vi "ORM Full Example.vi"() -> ()   [LabVIEW 2020, in "ORM_Examples.lvlib"]
uses:
  ORM_Examples.lvlib
  syslogs/syslogcluster.ctl
  syslogs/type.ctl
  <vilib>/Viviota/shared/ORM.lvlibp/ORM/SqlMapper/SqlMapper.lvclass
  <vilib>/Viviota/shared/ORM.lvlibp/ORM/TypeMap/TypeMap.lvclass
  syslogs/syslogs.lvclass
  syslogs/syslogs.lvclass/syslogs.ctl
  05764d67-500d-4b48-8229-7f30afda64a9.vi
  <vilib>/numeric/Random Number (Range) DBL.vi
  6377c067-cfd4-4b32-8915-bdbb0adddf30.vi
  0386ddb9-f275-45d1-b7b4-687382315ca8.vi
  9e31a9a6-021b-445f-b77c-036ae0c99ecd.vi
  80d51cb0-5371-4b91-9bea-091f0997292c.vi
  4f43362e-f8cc-419c-9351-c2ae03d92930.vi
  4ebe4bd5-e54f-48a5-86b4-46e7f1bb6f5a.vi
  0437fd30-8bf0-43ae-9868-d75e91ee3b4b.vi
  c0336298-bb8b-4fb9-a827-d7aab42547a5.vi
  syslogs/Write id.vi
  syslogs/Write type.vi
  b6464032-c044-4b29-b6c1-8ea3cc686848.vi
  98a8b6ed-17aa-439b-9f56-f47df0604604.vi
  05764d67-500d-4b48-8229-7f30afda64a9.vi/bd23ee19-7bd1-410a-a455-250ae7eff562.vi
  6377c067-cfd4-4b32-8915-bdbb0adddf30.vi/35b31214-e0d6-4ae0-b34c-13eba9df70db.vi
  6377c067-cfd4-4b32-8915-bdbb0adddf30.vi/2e8f1eab-5a58-47e6-9224-d0a2895e31fd.vi
  0386ddb9-f275-45d1-b7b4-687382315ca8.vi/35b31214-e0d6-4ae0-b34c-13eba9df70db.vi
  0386ddb9-f275-45d1-b7b4-687382315ca8.vi/2e8f1eab-5a58-47e6-9224-d0a2895e31fd.vi
  9e31a9a6-021b-445f-b77c-036ae0c99ecd.vi/a9ccc3c9-891a-4d80-8d4f-837bdef88ccd.vi
  9e31a9a6-021b-445f-b77c-036ae0c99ecd.vi/8216614f-f413-45b3-8111-14f8d0271ea5.vi
  9e31a9a6-021b-445f-b77c-036ae0c99ecd.vi/fc6a5c23-d21f-4d2c-895e-66da96fa9491.vi
  80d51cb0-5371-4b91-9bea-091f0997292c.vi/a9ccc3c9-891a-4d80-8d4f-837bdef88ccd.vi
  80d51cb0-5371-4b91-9bea-091f0997292c.vi/8216614f-f413-45b3-8111-14f8d0271ea5.vi
  80d51cb0-5371-4b91-9bea-091f0997292c.vi/fc6a5c23-d21f-4d2c-895e-66da96fa9491.vi
  4f43362e-f8cc-419c-9351-c2ae03d92930.vi/a9ccc3c9-891a-4d80-8d4f-837bdef88ccd.vi
  4f43362e-f8cc-419c-9351-c2ae03d92930.vi/8216614f-f413-45b3-8111-14f8d0271ea5.vi
  4f43362e-f8cc-419c-9351-c2ae03d92930.vi/fc6a5c23-d21f-4d2c-895e-66da96fa9491.vi
  4ebe4bd5-e54f-48a5-86b4-46e7f1bb6f5a.vi/ce8babb2-619c-4b95-b634-e027cd54a13e.vi
  4ebe4bd5-e54f-48a5-86b4-46e7f1bb6f5a.vi/383c36e0-7191-4c70-923d-4cc1411f3794.vi
  4ebe4bd5-e54f-48a5-86b4-46e7f1bb6f5a.vi/dcffdf9a-60b2-440f-af14-9d618c05381d.vi
  0437fd30-8bf0-43ae-9868-d75e91ee3b4b.vi/ce8babb2-619c-4b95-b634-e027cd54a13e.vi
  0437fd30-8bf0-43ae-9868-d75e91ee3b4b.vi/383c36e0-7191-4c70-923d-4cc1411f3794.vi
  0437fd30-8bf0-43ae-9868-d75e91ee3b4b.vi/dcffdf9a-60b2-440f-af14-9d618c05381d.vi
  c0336298-bb8b-4fb9-a827-d7aab42547a5.vi/ce8babb2-619c-4b95-b634-e027cd54a13e.vi
  c0336298-bb8b-4fb9-a827-d7aab42547a5.vi/383c36e0-7191-4c70-923d-4cc1411f3794.vi
  c0336298-bb8b-4fb9-a827-d7aab42547a5.vi/dcffdf9a-60b2-440f-af14-9d618c05381d.vi
  b6464032-c044-4b29-b6c1-8ea3cc686848.vi/93c2cd5d-a53a-4cc2-b8c3-9c3eef6598b6.vi
  98a8b6ed-17aa-439b-9f56-f47df0604604.vi/bd23ee19-7bd1-410a-a455-250ae7eff562.vi
  9e31a9a6-021b-445f-b77c-036ae0c99ecd.vi/fc6a5c23-d21f-4d2c-895e-66da96fa9491.vi/9d007ba8-e96f-4737-8d8a-6b46cf7f5c4a.vi
  9e31a9a6-021b-445f-b77c-036ae0c99ecd.vi/fc6a5c23-d21f-4d2c-895e-66da96fa9491.vi/050765a8-e5d4-4415-b637-62775228e838.vi
  80d51cb0-5371-4b91-9bea-091f0997292c.vi/fc6a5c23-d21f-4d2c-895e-66da96fa9491.vi/9d007ba8-e96f-4737-8d8a-6b46cf7f5c4a.vi
  80d51cb0-5371-4b91-9bea-091f0997292c.vi/fc6a5c23-d21f-4d2c-895e-66da96fa9491.vi/050765a8-e5d4-4415-b637-62775228e838.vi
  4f43362e-f8cc-419c-9351-c2ae03d92930.vi/fc6a5c23-d21f-4d2c-895e-66da96fa9491.vi/9d007ba8-e96f-4737-8d8a-6b46cf7f5c4a.vi
  4f43362e-f8cc-419c-9351-c2ae03d92930.vi/fc6a5c23-d21f-4d2c-895e-66da96fa9491.vi/050765a8-e5d4-4415-b637-62775228e838.vi
  <vilib>/Viviota/shared/ORM_ADONet.lvlibp/ADOMapper/ADOMapper.lvclass
  C:/Program Files/National Instruments/LabVIEW 2024/vi.lib/Viviota/shared/ORM.lvlibp/ORM/SqlMapper/SqlMapper.lvclass
  <vilib>/Viviota/shared/ORM.lvlibp/ORM/TypeMap/Write Autokey.vi
  <vilib>/Viviota/shared/ORM.lvlibp/ORM/TypeMap/Write Table Name.vi
  <vilib>/Viviota/shared/ORM_DBC_Sqlite.lvlibp/Sqlite Connect.vi
  <vilib>/Viviota/shared/ORM_DBC_Npgsql.lvlibp/Postgresql Connect.vi
  <vilib>/Viviota/shared/ORM_DBC_Mssql.lvlibp/SQL Connect.vi
  <vilib>/Utility/error.llb/Error Cluster From Error Code.vi
  <vilib>/Viviota/shared/ORM.lvlibp/ORM/TypeMap/Read TypeMap.vi
  <vilib>/Viviota/shared/ORM.lvlibp/ORM/SqlMapper/End Transaction.vi
  <vilib>/Viviota/shared/ORM.lvlibp/ORM/TypeMap/Where.vi
  <vilib>/Viviota/shared/ORM.lvlibp/ORM/Query Result/Next.vi
  <vilib>/Viviota/shared/ORM.lvlibp/ORM/TypeMap/ToLabVIEW_Wrap.vi
  <vilib>/Viviota/shared/ORM.lvlibp/ORM/DynamicParameters/DynamicParameters.lvclass
  <vilib>/Viviota/shared/ORM.lvlibp/ORM/Query Result/Query Result.lvclass
  ORM_API/ORM_API.lvlib
  <vilib>/Viviota/shared/ORM_ADONet.lvlibp
  <vilib>/Viviota/shared/ORM_DBC_Sqlite.lvlibp/DBC.lvclass
  <vilib>/Viviota/shared/ORM_DBC_Mssql.lvlibp/DBC.lvclass
  <vilib>/Viviota/shared/ORM_DBC_Npgsql.lvlibp/DBC.lvclass
  <vilib>/Viviota/shared/ORM.lvlibp/Transaction Logger/Log Map/LogMap.lvclass
  baf2aaaf-5c25-4d5a-81b7-a781a1585a2d.vi
  84ec28b1-c7a7-454f-ae3a-af914e71003c.vi
  50dc8464-3f00-4ac1-a87d-782bf5ccae4b.vi
  C:/Program Files/National Instruments/LabVIEW 2024/vi.lib/Viviota/shared/ORM_ADONet.lvlibp/ADOMapper/ADOMapper.lvclass
panel:
  out "DeleteTime":dbl
  in  "DeleteId":i32
  in  "DeleteEntry":bool
  out "QueryTime":dbl
  out "Count":i32
  out "ResultsTable":string
  out "Results":T1[](array[typedef]) {"Time Stamp" format="%<%x %.3X>T"}
  in  "limit":i32=10
  in  "ReturnAll":bool=TRUE
  in  "WHERE mode":enum32{"id", "type", "where"}(radio)=enum."type"
  in  "ExecuteQuery":bool
  in  "Explicit WHERE clause":string="executiontime < 4 AND executiontime > 2"
  in  "SyslogId":i32
  in  "SyslogType":string="warning"
  out "lastId":i32
  out "CreateTime":dbl
  in  "Use Bulk Create":bool=TRUE
  in  "Records":i32=100
  in  "PopulateTable":bool
  out "Error Out":errorcluster
  in  "Close":bool
  in  "DeleteTable":bool
  in  "CreateTable":bool
  in  "ConnectionString":string
  in  "SQLite Path":path
  in  "Connect":bool
  in  "DbType":string(combo)="Sqlite"
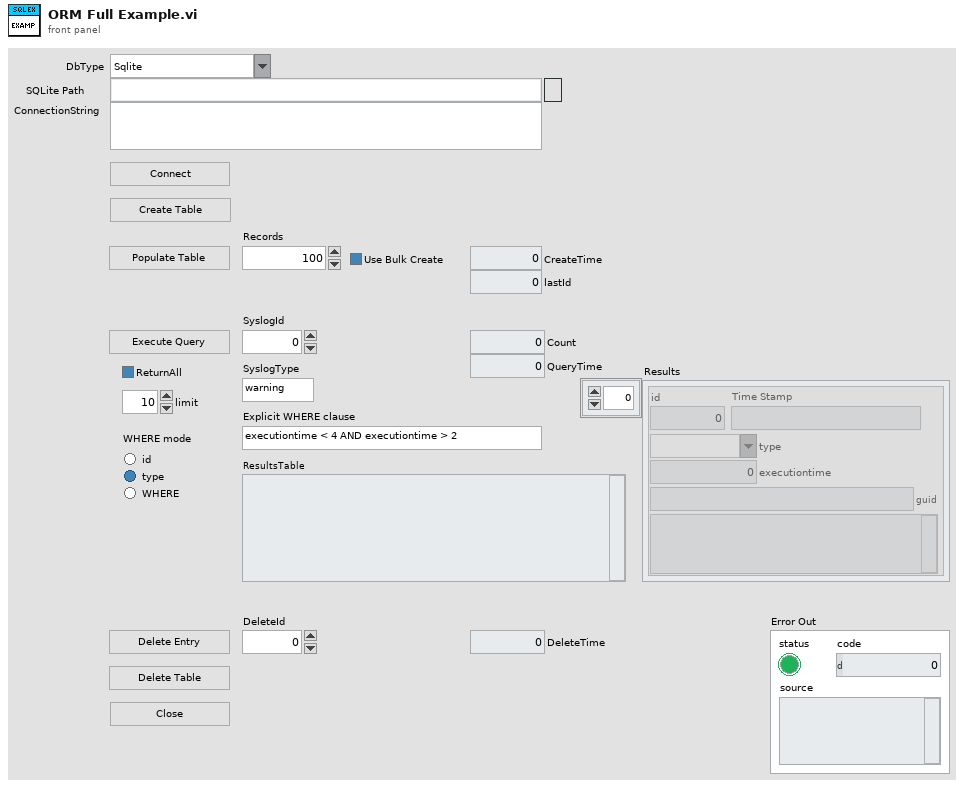
[diagram p1: front panel]
types:
  T1 = typedef "ORM_Examples.lvlib/syslogs.lvclass/syslogcluster.ctl" = cluster{"id":i32, "type":T2, "executiontime":dbl, "log":string, "guid":string, "Time Stamp":timestamp}
  T2 = typedef "ORM_Examples.lvlib/syslogs.lvclass/type.ctl" = string
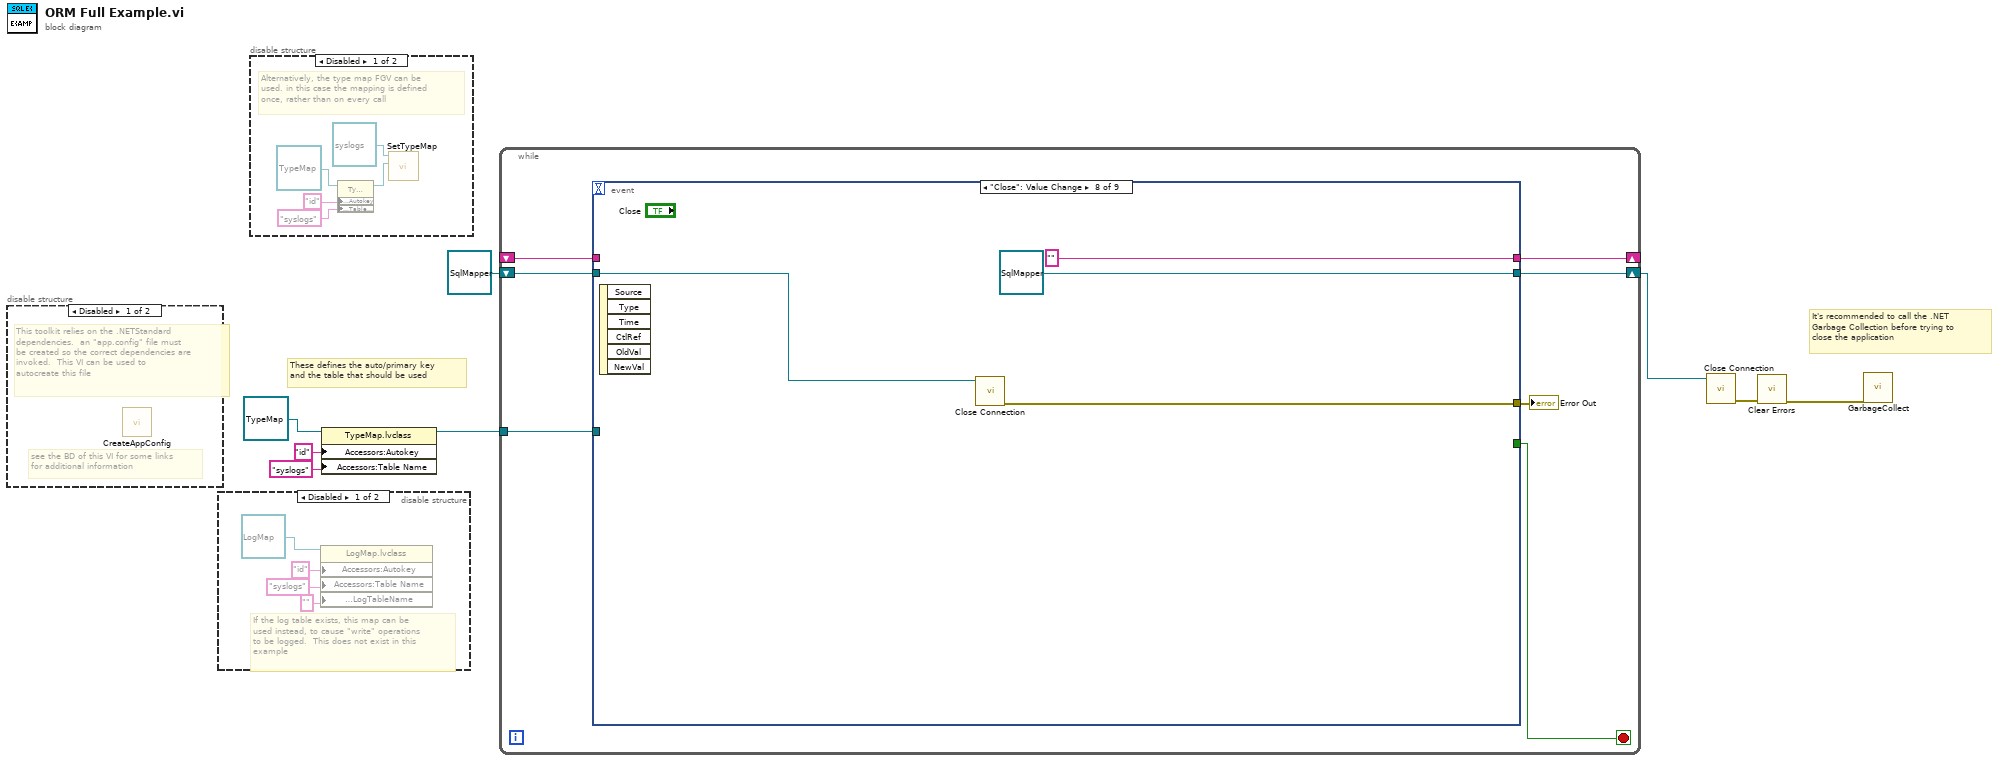
[diagram p0: block diagram]
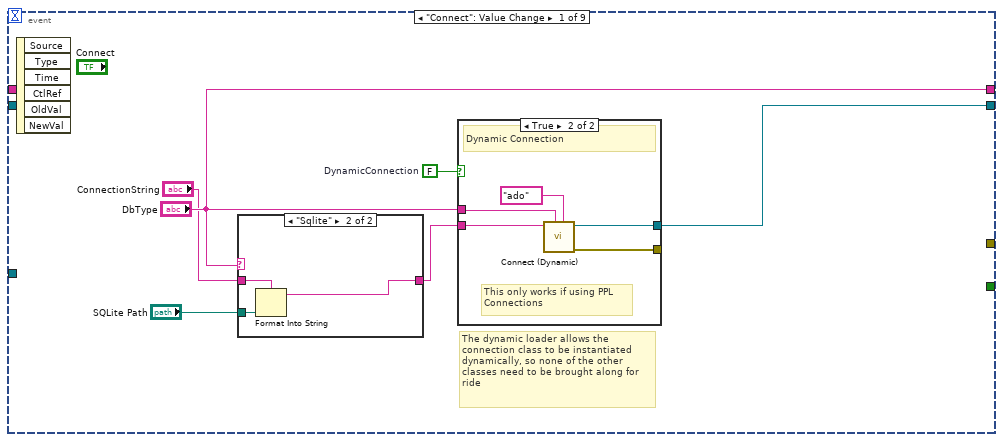
[diagram p5: hidden frame]
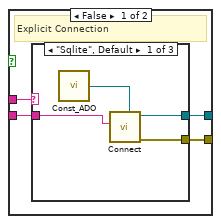
[diagram p7: hidden frame]
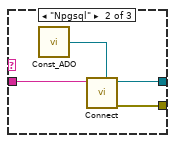
[diagram p8: hidden frame]
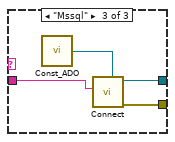
[diagram p9: hidden frame]
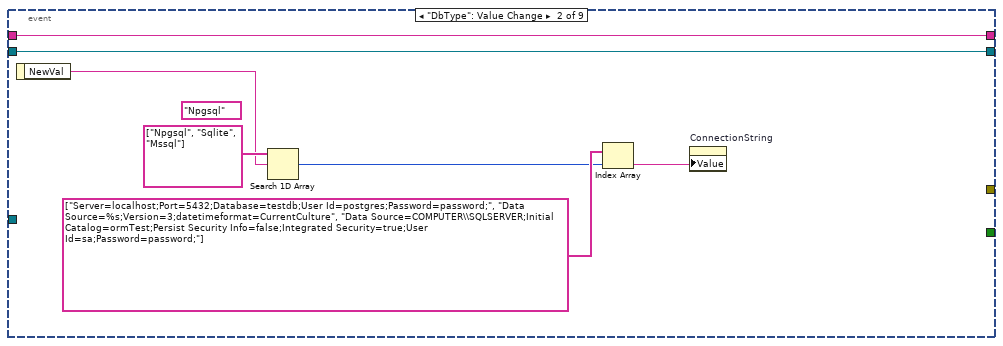
[diagram p10: hidden frame]
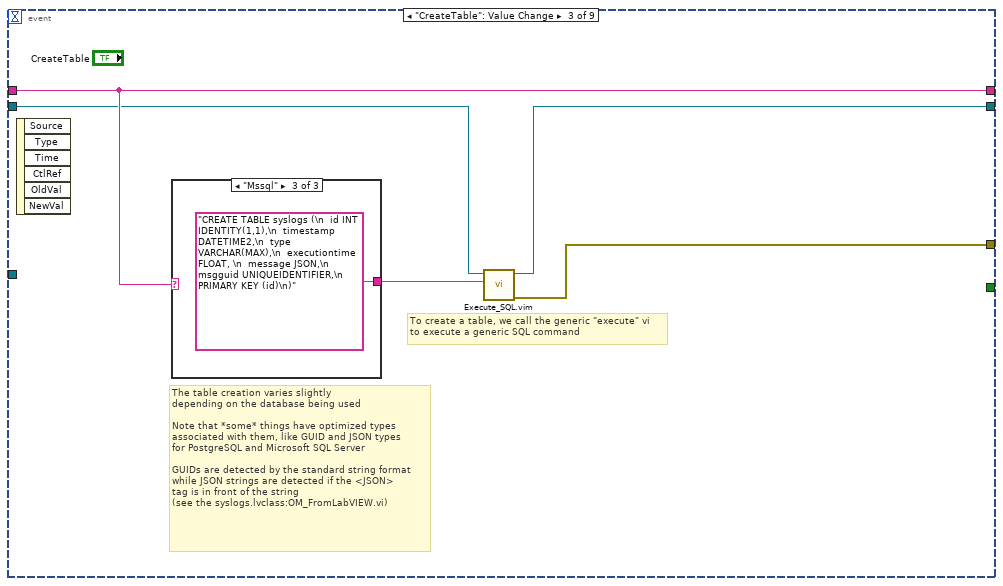
[diagram p11: hidden frame]
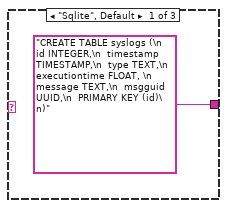
[diagram p12: hidden frame]
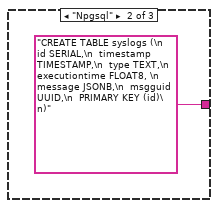
[diagram p13: hidden frame]
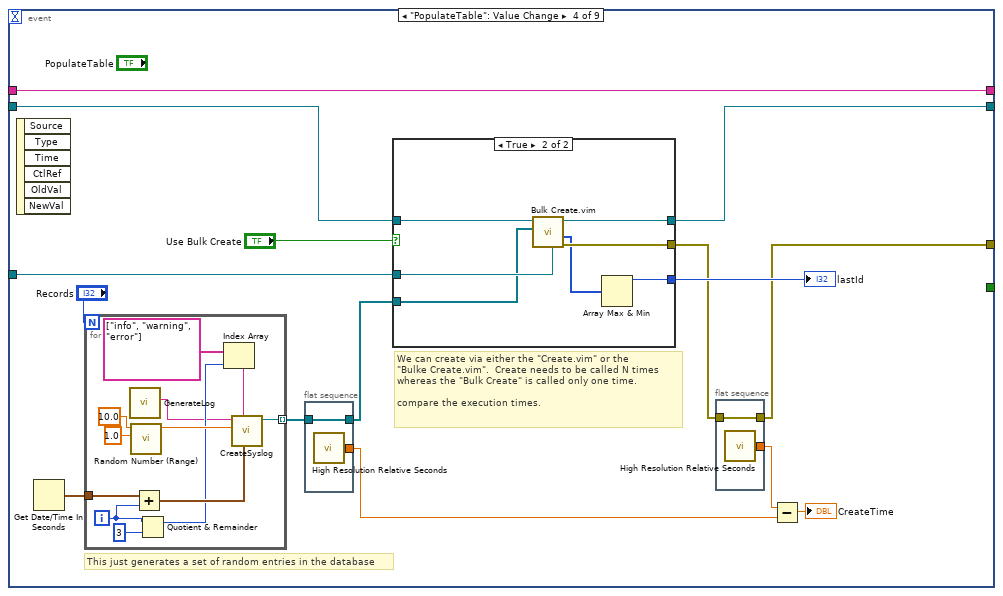
[diagram p14: hidden frame]
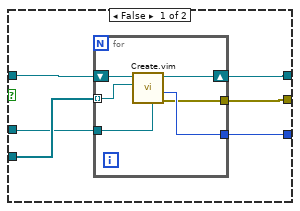
[diagram p15: hidden frame]
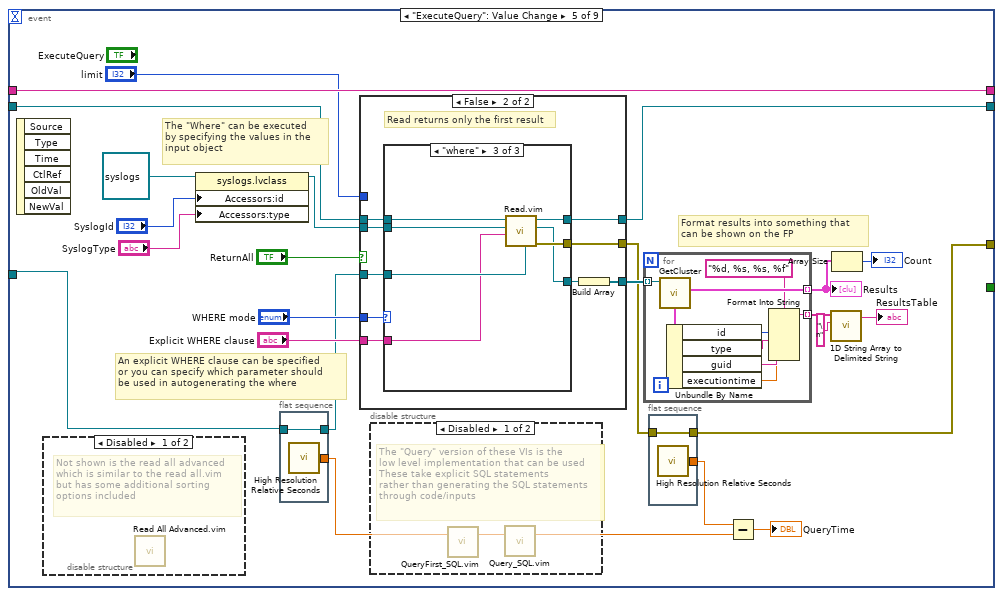
[diagram p16: hidden frame]
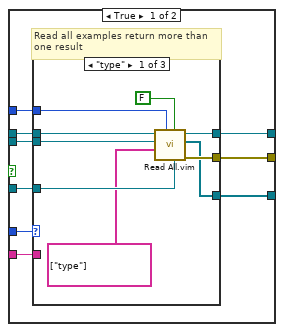
[diagram p19: hidden frame]
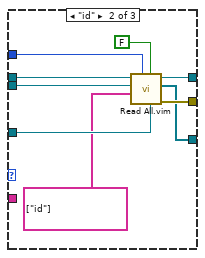
[diagram p20: hidden frame]
diagram:
  # "It's recommended to call the .NET \nGarbage Collection before trying to \nclose the application"
  # "These defines the auto/primary key\nand the table that should be used"
  n1 = disable-structure shown="Disabled" {
    frame Disabled {
      # "see the BD of this VI for some links\nfor additional information"
      # "This toolkit relies on the .NETStandard\ndependencies.  an \"app.config\" file must\nbe created so the correct dependencies are\ninvoked.  This VI can be used to \nautocreate this file"
      n2 = call "CreateAppConfig.vi"() -> ()  [unwired: 11 in, 1 out]
    }
    frame Enabled {
    }
  }
  n3 = disable-structure shown="Disabled" {
    frame Disabled {
      # "If the log table exists, this map can be\nused instead, to cause \"write\" operations\nto be logged.  This does not exist in this\nexample"
      n4 = property class="LogMap.lvclass"(reference=refnum<class "LogMap.lvclass"> refnum ("TypeMap in"), "Accessors:Autokey"="id" ("Autokey"), "Accessors:Table Name"="syslogs" ("Table Name"), "Data Member Access:LogTableName"="" ("LogTableName")) -> ()  [unwired: 1 in, 2 out]
    }
    frame Enabled {
    }
  }
  n5 = disable-structure shown="Disabled" {
    frame Disabled {
      # "Alternatively, the type map FGV can be\nused. in this case the mapping is defined\nonce, rather than on every call"
      n6 = property class="TypeMap.lvclass"(reference=refnum<class "TypeMap.lvclass"> refnum ("TypeMap in"), "Accessors:Autokey"="id" ("Autokey"), "Accessors:Table Name"="syslogs" ("Table Name")) -> (reference out=w14:refnum<class "TypeMap.lvclass">)  [unwired: 1 in, 1 out]
      n7 = call "SetTypeMap.vi"("TypeMap in"=w14, "object in"=refnum<class "syslogs.lvclass"> refnum ("ORM_Examples.lvlib:syslogs.lvclass")) -> ()  [unwired: 7 in, 3 out]
    }
    frame Enabled {
    }
  }
  n8 = property class="TypeMap.lvclass"(reference=refnum<class "TypeMap.lvclass"> refnum ("TypeMap in"), "Accessors:Autokey"="id" ("Autokey"), "Accessors:Table Name"="syslogs" ("Table Name")) -> (reference out=w4:refnum<class "TypeMap.lvclass">)  [unwired: 1 in, 1 out]
  n9 = while {
    shift-right: [w23] -> w3
    shift-left: refnum<class "SqlMapper.lvclass"> refnum ("SqlMapper out") -> [w22]
    shift-right: [w21] -> _
    shift-left: _ -> [w20]
    tunnel: w4 -> [w18]
    stop <- w24 stop-if-true
    n10 = event shown="[7] \"Close\": Value Change" {
      selector: _ -> [_ _ _ _ _ _ _ _ _]
      dyn-events: _ -> [_ _ _ _ _ _ _ _ _]
      timeout: _ -> [_ _ _ _ _ _ _ _ _]
      tunnel: [_ _ _ _ _ _ _ _ w251] -> w24
      tunnel: [w29 w56 w64 w82 w142 w233 w242 refnum<class "SqlMapper.lvclass"> refnum ("SqlMapper out") w249] -> w23
      tunnel: w22 -> [_ w56 w66 w83 w143 w234 w243 w246 w249]
      tunnel: ["DbType" w61 w67 w85 w144 w235 w244 "" ("DbType") w250] -> w21
      tunnel: w20 -> [_ w61 w67 w85 w144 w235 w244 _ w250]
      tunnel: [_ _ w63 w75 w126 w226 w241 w245 _] -> w19
      tunnel: w18 -> [_ _ _ w84 w125 w229 _ _ _]
      event "Connect": Value Change {
        w30 = FALSE  # DynamicConnection
        # "The dynamic loader allows the \nconnection class to be instantiated\ndynamically, so none of the other\nclasses need to be brought along for\nride"
        n11 = event-data() -> ()  [unwired: 1 in, 6 out]
        n12 = case shown="\"Sqlite\"" "DbType" {
          tunnel: "ConnectionString" -> [w31 w34]
          tunnel: "SQLite Path" -> [_ w33]
          tunnel: [w31 w32] -> w25
          frame "False", Default {
          }
          frame "Sqlite" {
            n13 = Format Into String(format string=w34, w33) -> (resulting string=w32:string)  [unwired: 2 in, 1 out]
          }
        }
        n14 = case shown="True" w30 {
          tunnel: "DbType" -> [w38 w53]
          tunnel: [w37 w55] -> w29
          tunnel: [w36 w54] -> _
          tunnel: w25 -> [w35 w51]
          frame False {
            # "Explicit Connection"
            n15 = case shown="\"Sqlite\", Default" w38 {
              tunnel: [w40 w44 w49] -> w37
              tunnel: [w41 w45 w48] -> w36
              tunnel: w35 -> [w39 w43 w47]
              frame "Sqlite", Default {
                n16 = call <vilib>:"Const_ADO.vi"() -> ("ADOMapper"=w42:refnum<class "ADOMapper.lvclass">)
                n17 = call-poly "Connect.vi"("SqlMapper Type"=w42, "Connection String"=w39) -> ("error out"=w41:errorcluster, "SqlMapper out"=w40:refnum<class "ADOMapper.lvclass">)  [unwired: 8 in]
              }
              frame "Npgsql" {
                n18 = call <vilib>:"Const_ADO.vi"() -> ("ADOMapper"=w46:refnum<class "ADOMapper.lvclass">)
                n19 = call-poly "Connect.vi"("SqlMapper Type"=w46, "Connection String"=w43) -> ("error out"=w45:errorcluster, "SqlMapper out"=w44:refnum<class "ADOMapper.lvclass">)  [unwired: 8 in]
              }
              frame "Mssql" {
                n20 = call <vilib>:"Const_ADO.vi"() -> ("ADOMapper"=w50:refnum<class "ADOMapper.lvclass">)
                n21 = call-poly "Connect.vi"("SqlMapper Type"=w50, "Connection String"=w47) -> ("error out"=w48:errorcluster, "SQL Mapper"=w49:refnum<class "ADOMapper.lvclass">)  [unwired: 8 in]
              }
            }
          }
          frame True {
            # "This only works if using PPL\nConnections"
            # "Dynamic Connection"
            n22 = call "Connect (Dynamic).vi"("SqlMapper"="ado", "DbType"=w53, "Connection String"=w51) -> ("error out"=w54:errorcluster, "SqlMapper out"=w55:refnum<class "SqlMapper.lvclass">)  [unwired: 7 in]
          }
        }
      }
      event "DbType": Value Change {
        (unwired) "Npgsql" ("DbType")
        n23 = event-data() -> ("NewVal"=w57:string)  [unwired: 1 in]
        n24 = Search 1D Array(1D array=string[] ["Npgsql", "Sqlite", "Mssql"], element=w57) -> (index of element=w59:i32)  [unwired: 1 in]
        n25 = Index Array(array=string[] ["Server=localhost;Port=5432;Database=testdb;User Id=postgres;Password=password;", "Data Source=%s;Version=3;datetimeformat=CurrentCulture", "Data Source=COMPUTER\\SQLSERVER;Initial Catalog=ormTest;Persist Security Info=false;Integrated Security=true;User Id=sa;Password=password;"], index=w59) -> (element=w58:string)
        n26 = property on="ConnectionString" class="Str"("Value"=w58) -> ()  [unwired: 2 in, 2 out]
      }
      event "CreateTable": Value Change {
        # "The table creation varies slightly\ndepending on the database being used\n\nNote that *some* things have optimized types\nassociated with them, like GUID and JSON types\nfor PostgreSQL and Microsoft SQL Server\n\nGUIDs are detected by the standard string format\nwhile JSON strings are detected if the <JSON>\ntag is in front of the string \n(see the syslogs.lvclass:OM_FromLabVIEW.vi)"
        # "To create a table, we call the generic \"execute\" vi\nto execute a generic SQL command"
        n27 = event-data() -> ()  [unwired: 1 in, 6 out]
        n28 = case shown="\"Mssql\"" w67 {
          tunnel: ["CREATE TABLE syslogs (\n  id INTEGER,\n  timestamp TIMESTAMP,\n  type TEXT,\n  executiontime FLOAT, \n  message TEXT,\n  msgguid UUID,\n  PRIMARY KEY (id)\n)" "CREATE TABLE syslogs (\n  id SERIAL,\n  timestamp TIMESTAMP,\n  type TEXT,\n  executiontime FLOAT8, \n  message JSONB,\n  msgguid UUID,\n  PRIMARY KEY (id)\n)" "CREATE TABLE syslogs (\n  id INT IDENTITY(1,1),\n  timestamp DATETIME2,\n  type VARCHAR(MAX),\n  executiontime FLOAT, \n  message JSON,\n  msgguid UNIQUEIDENTIFIER,\n  PRIMARY KEY (id)\n)"] -> w65
          frame "Sqlite", Default {
          }
          frame "Npgsql" {
          }
          frame "Mssql" {
          }
        }
        n29 = call "Execute_SQL.vim"("sql"=w65, "SqlMapper in"=w66) -> ("error out"=w63:errorcluster, "SqlMapper out"=w64:refnum<class "SqlMapper.lvclass">)  [unwired: 7 in, 1 out]
      }
      event "PopulateTable": Value Change {
        # "We can create via either the \"Create.vim\" or the \n\"Bulke Create.vim\".  Create needs to be called N times\nwhereas the \"Bulk Create\" is called only one time.\n\ncompare the execution times."
        # "This just generates a set of random entries in the database"
        n30 = event-data() -> ()  [unwired: 1 in, 6 out]
        n31 = Get Date/Time In Seconds() -> (seconds since 1Jan1904=w81:timestamp)
        n32 = for {
          N: "Records" -> [_]
          tunnel: [w101] -> w78 mode=indexing
          tunnel: w81 -> [w97]
          i -> [w95]
          n33 = call "GenerateLog.vi"() -> ("JSON"=w90:string)  [unwired: 10 in, 1 out]
          n34 = call-poly <vilib>:"Random Number (Range).vi"("lower bound (0)"=1.0, "upper bound (100)"=10.0) -> ("number"=w98:dbl)  [unwired: 9 in]
          n35 = Add(x=w97, y=w95) -> (x+y=w96:timestamp)
          n36 = Quotient & Remainder(x=w95, y=3) -> (x-y*floor(x/y)=w92:i32)  [unwired: 1 out]
          n37 = Index Array(array=T2[] ["info", "warning", "error"] ("Array"), index=w92) -> (element=w91:T2)
          n38 = call "CreateSyslog.vi"("timestamp"=w96, "type"=w91, "executiontime"=w98, "log"=w90) -> ("syslog out"=w101:refnum<class "syslogs.lvclass">)  [unwired: 6 in, 1 out]
        }
        n39 = flat-sequence {
          tunnel: [w89] -> w73
          tunnel: w78 -> [w88]
          tunnel: [w88] -> w77
          frame #0 {
            n40 = call <vilib>:"High Resolution Relative Seconds.vi"() -> ("relative seconds"=w89:dbl)
          }
        }
        n41 = case shown="True" "Use Bulk Create" {
          tunnel: w84 -> [w102 w120]
          tunnel: [w104 w119] -> w76
          tunnel: w83 -> [w107 w118]
          tunnel: [w106 w117] -> w82
          tunnel: w77 -> [w103 w116]
          tunnel: [w105 w114] -> w80
          frame False {
            n42 = for {
              tunnel: [w111] -> w105
              tunnel: [w110] -> w104
              shift-right: [w112] -> w106
              shift-left: w107 -> [w113]
              tunnel: w103 -> [w109] mode=indexing
              tunnel: w102 -> [w108]
              n43 = call "Create.vim"("TypeMap in"=w108, "object in"=w109, "SqlMapper in"=w113) -> ("error out"=w110:errorcluster, "id"=w111:i32, "SqlMapper out"=w112:refnum<class "SqlMapper.lvclass">)  [unwired: 5 in, 1 out]
            }
          }
          frame True {
            n44 = call "Bulk Create.vim"("TypeMap in"=w120, "object in"=w116, "SqlMapper in"=w118) -> ("error out"=w119:errorcluster, "id"=w115:i32[], "SqlMapper out"=w117:refnum<class "SqlMapper.lvclass">)  [unwired: 5 in, 1 out]
            n45 = Array Max & Min(array=w115) -> (max value=w114:i32)  [unwired: 3 out]
          }
        }
        "lastId" <- w80
        n46 = flat-sequence {
          tunnel: [w87] -> w74
          tunnel: w76 -> [w86]
          tunnel: [w86] -> w75
          frame #0 {
            n47 = call <vilib>:"High Resolution Relative Seconds.vi"() -> ("relative seconds"=w87:dbl)
          }
        }
        n48 = Subtract(x=w74, y=w73) -> (x-y=→"CreateTime":dbl)
      }
      event "ExecuteQuery": Value Change {
        # "An explicit WHERE clause can be specified\nor you can specify which parameter should\nbe used in autogenerating the where"
        # "The \"Where\" can be executed\nby specifying the values in the \ninput object"
        # "Format results into something that \ncan be shown on the FP"
        n49 = event-data() -> ()  [unwired: 1 in, 6 out]
        n50 = disable-structure shown="Disabled" {
          frame Disabled {
            # "Not shown is the read all advanced\nwhich is similar to the read all.vim\nbut has some additional sorting\noptions included"
            n51 = call "Read All Advanced.vim"() -> ()  [unwired: 9 in, 3 out]
          }
          frame Enabled {
          }
        }
        n52 = property class="syslogs.lvclass"(reference=refnum<class "syslogs.lvclass"> refnum ("ORM_Examples.lvlib:syslogs.lvclass"), "Accessors:id"="SyslogId", "Accessors:type"="SyslogType") -> (reference out=w139:refnum<class "syslogs.lvclass">)  [unwired: 1 in, 1 out]
        n53 = flat-sequence {
          tunnel: [w148] -> w123
          tunnel: w125 -> [w147]
          tunnel: [w147] -> w124
          frame #0 {
            n54 = call <vilib>:"High Resolution Relative Seconds.vi"() -> ("relative seconds"=w148:dbl)
          }
        }
        n55 = case shown="False" "ReturnAll" {
          tunnel: w143 -> [w165 w201]
          tunnel: [w164 w200] -> w142
          tunnel: w124 -> [w163 w199]
          tunnel: [w162 w198] -> w127
          tunnel: "WHERE mode" -> [w161 w197]
          tunnel: w139 -> [w160 w196]
          tunnel: "Explicit WHERE clause" -> [w159 w195]
          tunnel: "limit" -> [w158 _]
          tunnel: [w157 w193] -> w134
          frame True {
            # "Read all examples return more than\none result"
            n56 = case shown="\"type\"" w161 {
              tunnel: w165 -> [w174 w183 w192]
              tunnel: [w173 w182 w191] -> w164
              tunnel: w163 -> [w172 w181 w190]
              tunnel: [w171 w180 w189] -> w162
              tunnel: w160 -> [w170 w179 w188]
              tunnel: w159 -> [_ _ w187]
              tunnel: [w168 w177 w186] -> w157
              tunnel: w158 -> [w167 w176 w185]
              frame "type" {
                n57 = call "Read All.vim"("TypeMap in"=w172, "Select All"=FALSE, "Limit"=w167, "WHERE"=string[] ["type"], "Object"=w170, "SqlMapper in"=w174) -> ("error out"=w171:errorcluster, "Query Results"=w168:refnum<class "syslogs.lvclass">[], "SqlMapper out"=w173:refnum<class "SqlMapper.lvclass">)  [unwired: 3 in]
              }
              frame "id" {
                n58 = call "Read All.vim"("TypeMap in"=w181, "Select All"=FALSE, "Limit"=w176, "WHERE"=string[] ["id"], "Object"=w179, "SqlMapper in"=w183) -> ("error out"=w180:errorcluster, "Query Results"=w177:refnum<class "syslogs.lvclass">[], "SqlMapper out"=w182:refnum<class "SqlMapper.lvclass">)  [unwired: 3 in]
              }
              frame "where" {
                n59 = call "Read All.vim"("TypeMap in"=w190, "Select All"=FALSE, "Limit"=w185, "WHERE"=w187, "Object"=w188, "SqlMapper in"=w192) -> ("error out"=w189:errorcluster, "Query Results"=w186:refnum<class "syslogs.lvclass">[], "SqlMapper out"=w191:refnum<class "SqlMapper.lvclass">)  [unwired: 3 in]
              }
            }
          }
          frame False {
            # "Read returns only the first result"
            n60 = case shown="\"where\"" w197 {
              tunnel: w201 -> [w208 w215 w222]
              tunnel: [w207 w214 w221] -> w200
              tunnel: w199 -> [w206 w213 w220]
              tunnel: [w205 w212 w219] -> w198
              tunnel: w196 -> [w204 w211 w218]
              tunnel: w195 -> [_ _ w217]
              tunnel: [w202 w209 w216] -> w194
              frame "type" {
                n61 = call "Read.vim"("TypeMap in"=w206, "Where"=string[] ["type"], "object in"=w204, "SqlMapper in"=w208) -> ("error out"=w205:errorcluster, "object out"=w202:refnum<class "syslogs.lvclass">, "SqlMapper out"=w207:refnum<class "SqlMapper.lvclass">)  [unwired: 4 in, 1 out]
              }
              frame "id" {
                n62 = call "Read.vim"("TypeMap in"=w213, "Where"=string[] ["id"], "object in"=w211, "SqlMapper in"=w215) -> ("error out"=w212:errorcluster, "object out"=w209:refnum<class "syslogs.lvclass">, "SqlMapper out"=w214:refnum<class "SqlMapper.lvclass">)  [unwired: 4 in, 1 out]
              }
              frame "where" {
                n63 = call "Read.vim"("TypeMap in"=w220, "Where"=w217, "object in"=w218, "SqlMapper in"=w222) -> ("error out"=w219:errorcluster, "object out"=w216:refnum<class "syslogs.lvclass">, "SqlMapper out"=w221:refnum<class "SqlMapper.lvclass">)  [unwired: 4 in, 1 out]
              }
            }
            n64 = Build Array(w194) -> (w193:refnum<class "syslogs.lvclass">[])
          }
        }
        n65 = disable-structure shown="Disabled" {
          frame Disabled {
            # "The \"Query\" version of these VIs is the\nlow level implementation that can be used\nThese take explicit SQL statements\nrather than generating the SQL statements\nthrough code/inputs"
            n66 = call "QueryFirst_SQL.vim"() -> ()  [unwired: 9 in, 3 out]
            n67 = call "Query_SQL.vim"() -> ()  [unwired: 9 in, 3 out]
          }
          frame Enabled {
          }
        }
        n68 = for {
          tunnel: w134 -> [w156] mode=indexing
          tunnel: [w155] -> w129 mode=indexing
          tunnel: [w150] -> w133 mode=indexing
          n69 = call "GetCluster.vi"("syslogs in"=w156) -> ("Value"=w155:T1)  [unwired: 8 in, 2 out]
          n70 = Unbundle By Name(w155) -> ("id"=w154:i32, "type"=w153:T2, "guid"=w152:string, "executiontime"=w149:dbl)
          n71 = Format Into String(format string="%d, %s, %s, %f", w154, w153, w152, w149) -> (resulting string=w150:string)  [unwired: 2 in, 1 out]
        }
        "Results" <- w129
        n72 = flat-sequence {
          tunnel: [w146] -> w122
          tunnel: w127 -> [w145]
          tunnel: [w145] -> w126
          frame #0 {
            n73 = call <vilib>:"High Resolution Relative Seconds.vi"() -> ("relative seconds"=w146:dbl)
          }
        }
        n74 = Subtract(x=w122, y=w123) -> (x-y=→"QueryTime":dbl)
        n75 = call <vilib>:"1D String Array to Delimited String.vi"("delimiter"="\n", "string array"=w133) -> ("delimited string"=→"ResultsTable":string)  [unwired: 9 in]
        n76 = Array Size(array=w129) -> (size(s)=→"Count":i32)
      }
      event "DeleteEntry": Value Change {
        # "The Delete ONLY works\nusing the Autokey ID values\n\nFor more complex delete operations\nthe Execute_SQL.vim should be used"
        n77 = event-data() -> ()  [unwired: 1 in, 6 out]
        n78 = property class="syslogs.lvclass"(reference=refnum<class "syslogs.lvclass"> refnum ("ORM_Examples.lvlib:syslogs.lvclass"), "Accessors:id"="DeleteId") -> (reference out=w230:refnum<class "syslogs.lvclass">)  [unwired: 1 in, 1 out]
        n79 = flat-sequence {
          tunnel: [w239] -> w224
          tunnel: w229 -> [w238]
          tunnel: [w238] -> w228
          frame #0 {
            n80 = call <vilib>:"High Resolution Relative Seconds.vi"() -> ("relative seconds"=w239:dbl)
          }
        }
        n81 = call "Delete.vim"("TypeMap in"=w228, "object in"=w230, "SqlMapper in"=w234) -> ("error out"=w227:errorcluster, "SqlMapper out"=w233:refnum<class "SqlMapper.lvclass">)  [unwired: 6 in, 1 out]
        n82 = flat-sequence {
          tunnel: [w237] -> w225
          tunnel: w227 -> [w236]
          tunnel: [w236] -> w226
          frame #0 {
            n83 = call <vilib>:"High Resolution Relative Seconds.vi"() -> ("relative seconds"=w237:dbl)
          }
        }
        n84 = Subtract(x=w225, y=w224) -> (x-y=→"DeleteTime":dbl)
      }
      event "DeleteTable": Value Change {
        # "Deletes table using the explicit \"Execute\" VI"
        n85 = event-data() -> ()  [unwired: 1 in, 6 out]
        n86 = call "Execute_SQL.vim"("sql"="DROP TABLE syslogs", "SqlMapper in"=w243) -> ("error out"=w241:errorcluster, "SqlMapper out"=w242:refnum<class "SqlMapper.lvclass">)  [unwired: 7 in, 1 out]
      }
      event "Close": Value Change {
        n87 = event-data() -> ()  [unwired: 1 in, 6 out]
        n88 = call "Close Connection.vi"("SqlMapper"=w246) -> ("Error Out"=w245:errorcluster)  [unwired: 10 in]
      }
      event Panel Close? {
        w251 = TRUE ("Discard?")
        n89 = event-data() -> ()  [unwired: 1 in, 4 out]
        n90 = event-data("Discard?"=w251) -> ()  [unwired: 1 in, 1 out]
      }
    }
    "Error Out" <- w19
  }
  n91 = call "Close Connection.vi"("SqlMapper"=w3) -> ("Error Out"=w2:errorcluster)  [unwired: 10 in]
  n92 = call <vilib>:"Clear Errors.vi"("error in (no error)"=w2) -> ("error out"=w1:errorcluster)  [unwired: 5 in, 1 out]
  n93 = call "GarbageCollect.vi"("error in"=w1) -> ()  [unwired: 10 in, 1 out]
